vi "read_mask_from_file.vi"(8 "Error In":errorcluster, 9 "Sample":string, 10 "File Path":path, 11 "Image":T1) -> (0 "Error Out":errorcluster, 2 "data":T2 {"Contours"."Type" items=["No Selection", "Point", "Line", "Rectangle", "Oval", "Polygon", "Freehand Region", "Annulus", "Unused2", "Unused3", "Broken Line", "Freehand Line", "Rotated Rectangle"]}, 3 "Image Out":T1)   [LabVIEW 2019]
uses:
  <vilib>/vision/Image Controls.llb/IMAQ Image.ctl
  <vilib>/vision/NI_Vision_Development_Module.lvlib
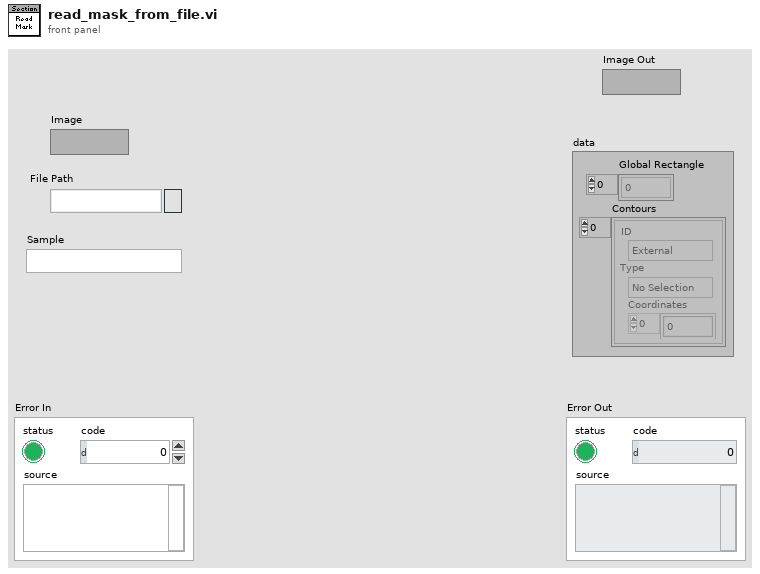
[diagram p1: front panel]
types:
  T1 = typedef "IMAQ Image.ctl" = refnum<image>
  T2 = typedef "ROI Descriptor" = cluster{"Global Rectangle":i32[], "Contours":cluster{"ID":enum32{"External", "Internal"}, "Type":u32, "Coordinates":i32[]}[]}
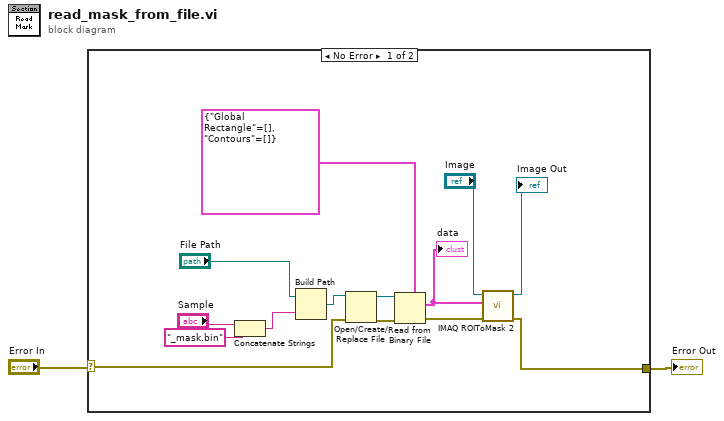
[diagram p0: block diagram]
diagram:
  n1 = case shown="No Error" "Error In" {
    selector: "Error In" -> [w4 w17]
    tunnel: [w3 w17] -> w1
    frame No Error {
      n2 = Concatenate Strings("Sample", "_mask.bin" ("string")) -> (w14:string)
      n3 = Build Path(base path="File Path", name or relative path=w14) -> (appended path=w12:path)
      n4 = Open/Create/Replace File(file path (use dialog)=w12, error in=w4) -> (refnum out=w11:refnum<file>, error out=w5:errorcluster)  [unwired: 4 in, 1 out]
      n5 = Read from Binary File(5:T2 {"Global Rectangle"=[], "Contours"=[]} ("ROI Descriptor Out"), 8:w5, 11:w11) -> (0:w6:errorcluster, 2:w9:T2)  [unwired: 3 in, 2 out]
      "data" <- w9
      n6 = call "IMAQ ROIToMask 2"("error in (no error)"=w6, "ROI Descriptor"=w9, "Image"="Image") -> ("error out"=w3:errorcluster, "Image Out"=→"Image Out":T1)  [unwired: 6 in, 1 out]
    }
    frame Error {
    }
  }
  "Error Out" <- w1
